vi "Delete Reference.vi"(0 "All Descendents":refnum<vi>[](array[refnum]), 5 "Numeric":i32, 11 "error in (no error)":errorcluster) -> (15 "error out":errorcluster)   [LabVIEW 2021, in "Migrator.lvlib"]
uses:
  Migrator.lvlib
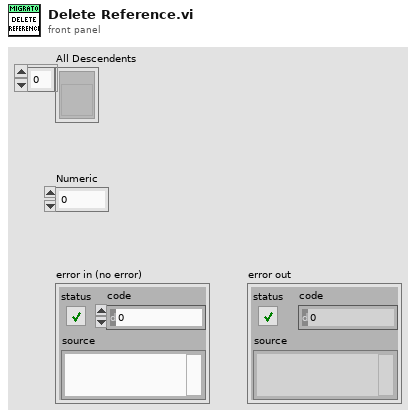
[diagram p1: front panel]
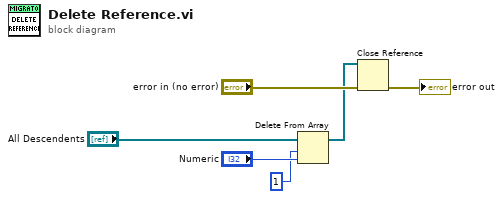
[diagram p0: block diagram]
diagram:
  n1 = Delete From Array(array="All Descendents", length=1, index="Numeric") -> (array with subset deleted=w4:refnum<vi>[])  [unwired: 1 out]
  n2 = Close Reference(reference=w4, error in (no error)="error in (no error)") -> (error out=→"error out":errorcluster)
